vi "scaling_calculator_baratron.vi"(2 "x":dbl, 3 "offset subt":dbl) -> (5 "y (Pa)":dbl, 6 "y (mTorr)":dbl)   [LabVIEW 2017]
uses:
  <vilib>/express/express arith-compare/Formula/XNode/ExpressFormulaBlockNode.xnode
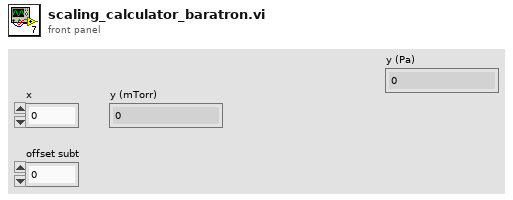
[diagram p1: front panel]
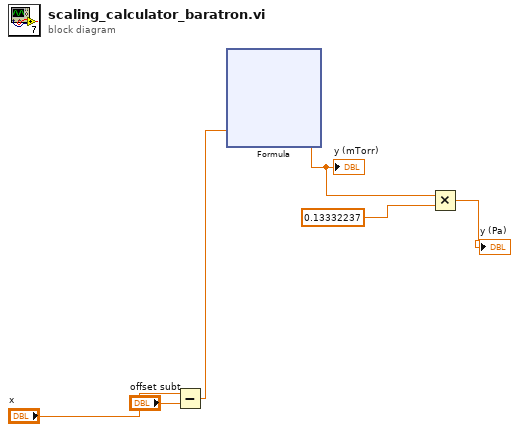
[diagram p0: block diagram]
diagram:
  n1 = Subtract(x="x", y="offset subt") -> (x-y=w1:dbl)
  n2 = xnode "Formula"("X"=w1) -> ("結果"=w5:dbl)  [unwired: 1 in, 1 out]
  "y (mTorr)" <- w5
  n3 = Multiply(x=w5, y=0.13332237) -> (x*y=→"y (Pa)":dbl)
